vi "Write lastUpdateTime.vi"(8 "error in (no error)":errorcluster, 10 "lastUpdateTime":dbl, 11 "SpectrographHeartbeat in":refnum<class "SpectrographHeartbeat.lvclass">) -> (0 "error out":errorcluster, 3 "SpectrographHeartbeat out":refnum<class "SpectrographHeartbeat.lvclass">)   [LabVIEW 2016, in "SpectrographHeartbeat.lvclass"]
uses:
  SpectrographHeartbeat.lvclass
  SpectrographHeartbeat.lvclass/SpectrographHeartbeat.ctl
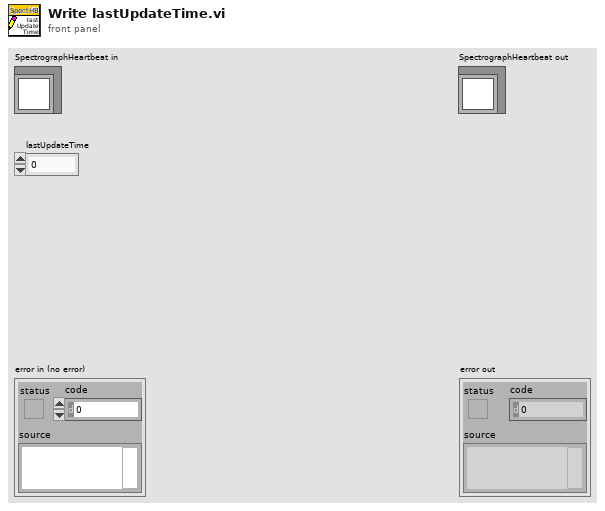
[diagram p1: front panel]
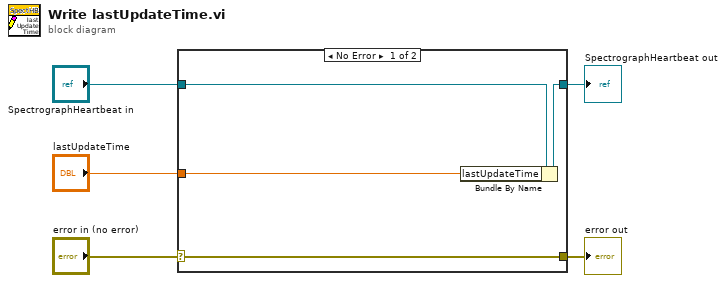
[diagram p0: block diagram]
diagram:
  n1 = case shown="No Error" "error in (no error)" {
    selector: "error in (no error)" -> [w9 w10]
    tunnel: [w9 w10] -> w4
    tunnel: [w7 w11] -> w2
    tunnel: "SpectrographHeartbeat in" -> [w8 w11]
    tunnel: "lastUpdateTime" -> [w6 _]
    frame No Error {
      n2 = Bundle By Name(cluster=w8, "lastUpdateTime"=w6) -> (w7:refnum<class "SpectrographHeartbeat.lvclass">)
    }
    frame Error {
    }
  }
  "error out" <- w4
  "SpectrographHeartbeat out" <- w2
